vi "Program10.vi"() -> ()   [LabVIEW 2020]
panel:
  out "LED 2":bool
  out "LED1":bool
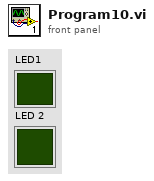
[diagram p1: front panel]
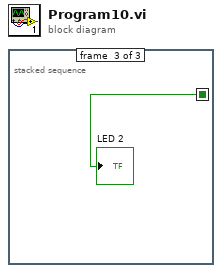
[diagram p0: block diagram]
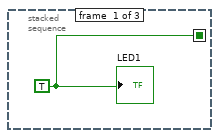
[diagram p2: hidden frame]
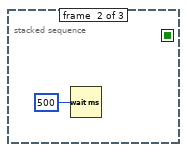
[diagram p3: hidden frame]
diagram:
  n1 = stacked-sequence {
    seq-local: [w1 _ _] -> [_ w2 _]
    seq-local: [_ w2 _] -> [_ _ w4]
    frame #0 {
      w1 = TRUE
      "LED1" <- w1
    }
    frame #1 {
      n2 = Wait (ms)(milliseconds to wait=u32 500) -> ()  [unwired: 1 out]
    }
    frame #2 {
      "LED 2" <- w4
    }
  }
